vi "Wrapper.vi"(0 "measurement configuration":T1={"Calculate Analysis?"=TRUE, "Current Setpoint"=1.2, "Voltage Setpoint"=0.0, "Physical Channel"="Lorem ipsum dolor sit"}, 5 "Physical Channel":tag="PowerModule/power", 11 "error in":errorcluster) -> (4 "measurement results":T2, 15 "error out":errorcluster)   [LabVIEW 2021, in "Z Power Module.lvlib"]
uses:
  Z Power Module.lvlib
  Measurement Results.ctl
  Measurement Configuration.ctl
  MeasurementCore/Main Library_Z Power Module.lvlib
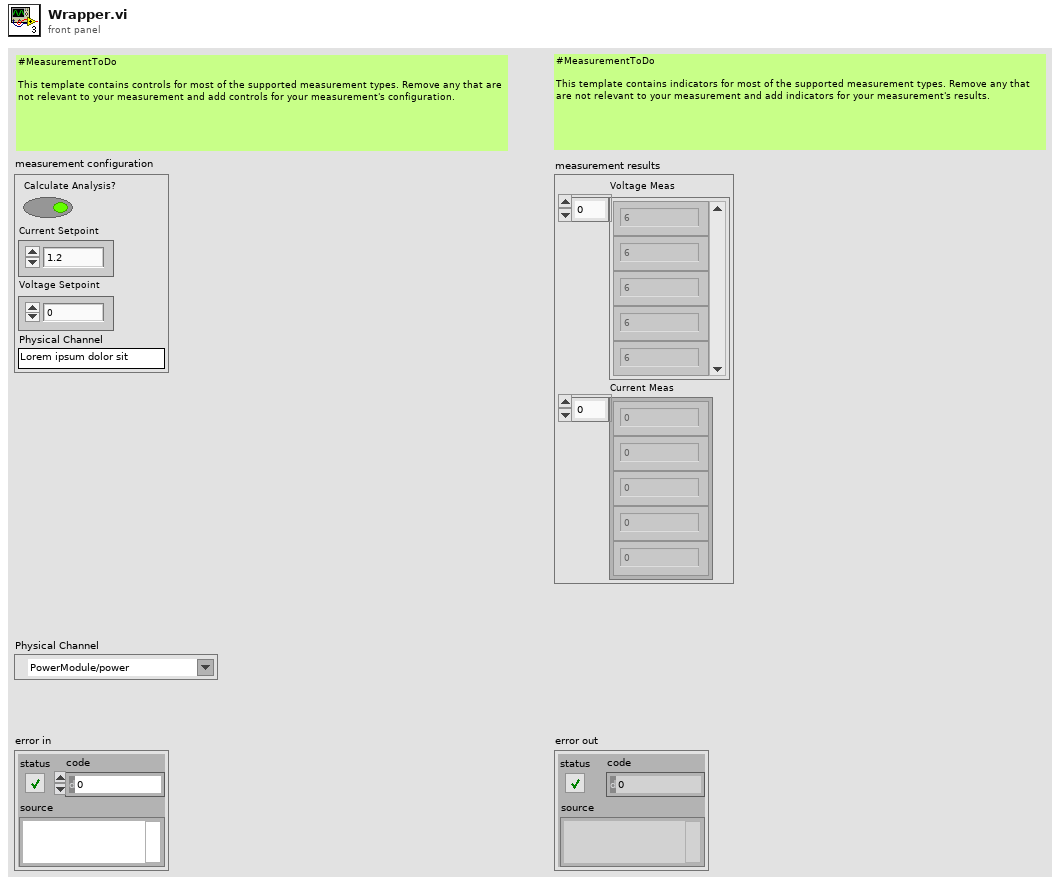
[diagram p1: front panel]
types:
  T1 = typedef "Z Power Module.lvlib/Measurement Configuration.ctl" = cluster{"Calculate Analysis?":bool, "Current Setpoint":dbl, "Voltage Setpoint":dbl, "Physical Channel":string}
  T2 = typedef "Z Power Module.lvlib/Measurement Results.ctl" = cluster{"Voltage Meas":dbl[], "Current Meas":dbl[]}
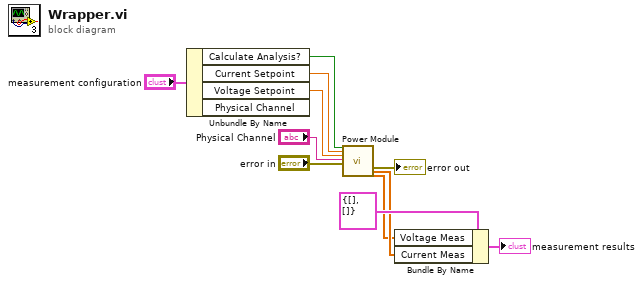
[diagram p0: block diagram]
diagram:
  n1 = Unbundle By Name("measurement configuration") -> ("Calculate Analysis?"=w5:bool, "Current Setpoint"=w4:dbl, "Voltage Setpoint"=w3:dbl)  [unwired: 1 out]
  n2 = call "Power Module.vi"("Calculate Analysis?"=w5, "Current Setpoint"=w4, "Voltage Setpoint"=w3, "Physical Channel"="Physical Channel", "error in"="error in") -> ("error out"=→"error out":errorcluster, "Current Meas"=w9:dbl[], "Voltage Meas"=w8:dbl[])  [unwired: 20 in]
  n3 = Bundle By Name(cluster=T2 {"Voltage Meas"=[], "Current Meas"=[]} ("measurement results"), "Voltage Meas"=w8, "Current Meas"=w9) -> (→"measurement results":T2)
